vi "Poly.vi"() -> ()   [LabVIEW 2020]
panel:
  out "Write ADAS Data":T1(array[cluster])
  out "Serialize ADAS Data":T1(array[cluster])
  out "Read ADAS Data":T1(array[cluster])
  out "Deserialize ADAS Data":T1(array[cluster])
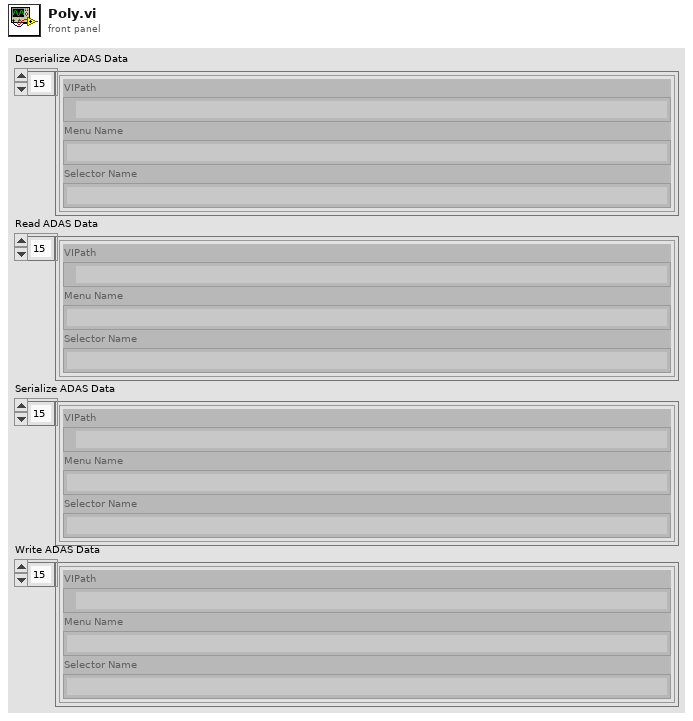
[diagram p1: front panel]
types:
  T1 = cluster{"VIPath":path, "Menu Name":string, "Selector Name":string}[]
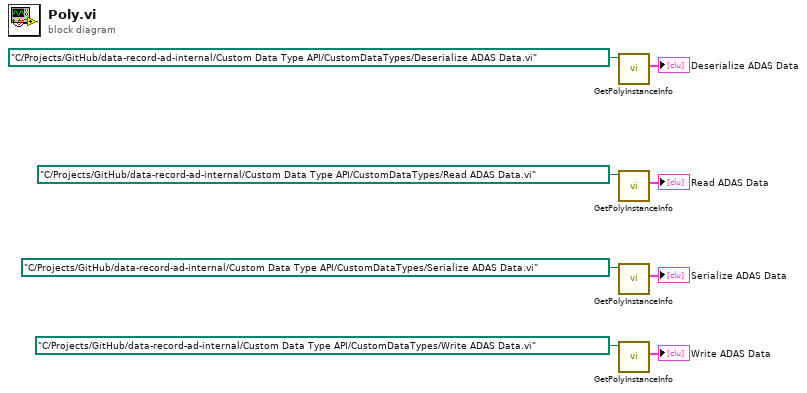
[diagram p0: block diagram]
diagram:
  n1 = call "GetPolyInstanceInfo.vi"("Poly VI Path"=path "C:/Projects/GitHub/data-record-ad-internal/Custom Data Type API/CustomDataTypes/Deserialize ADAS Data.vi") -> ("InstanceInfo"=→"Deserialize ADAS Data":T1)  [unwired: 8 in, 2 out]
  n2 = call "GetPolyInstanceInfo.vi"("Poly VI Path"=path "C:/Projects/GitHub/data-record-ad-internal/Custom Data Type API/CustomDataTypes/Read ADAS Data.vi") -> ("InstanceInfo"=→"Read ADAS Data":T1)  [unwired: 8 in, 2 out]
  n3 = call "GetPolyInstanceInfo.vi"("Poly VI Path"=path "C:/Projects/GitHub/data-record-ad-internal/Custom Data Type API/CustomDataTypes/Serialize ADAS Data.vi") -> ("InstanceInfo"=→"Serialize ADAS Data":T1)  [unwired: 8 in, 2 out]
  n4 = call "GetPolyInstanceInfo.vi"("Poly VI Path"=path "C:/Projects/GitHub/data-record-ad-internal/Custom Data Type API/CustomDataTypes/Write ADAS Data.vi") -> ("InstanceInfo"=→"Write ADAS Data":T1)  [unwired: 8 in, 2 out]
